vi "getIntersectionFromBallVelocityAndGoalLine.vi"(8 "error in (no error)":errorcluster, 11 "Utilities in":refnum<class "Utilities.lvclass">) -> (0 "error out":errorcluster, 3 "Utilities out":refnum<class "Utilities.lvclass">)   [LabVIEW 2023, in "Utilities.lvclass"]
uses:
  Utilities.lvclass
  Game_class/Game.lvclass
  Game_class/Game.lvclass/Game.ctl
  Ball_class/Ball.lvclass/Ball.ctl
  Object_class/Object.lvclass/Object.ctl
  Game_class/Read BallRef.vi
  Game_class/Read FieldRef.vi
  Ball_class/Read v_x.vi
  Ball_class/Read v_y.vi
  Object_class/Read x.vi
  Object_class/Read y.vi
  Ball_class/Ball.lvclass
  Field_class/Field.lvclass
panel:
  out "y_intersection":dbl
  out "x_intersection":dbl
  in  "Game":refnum<class "Game.lvclass">
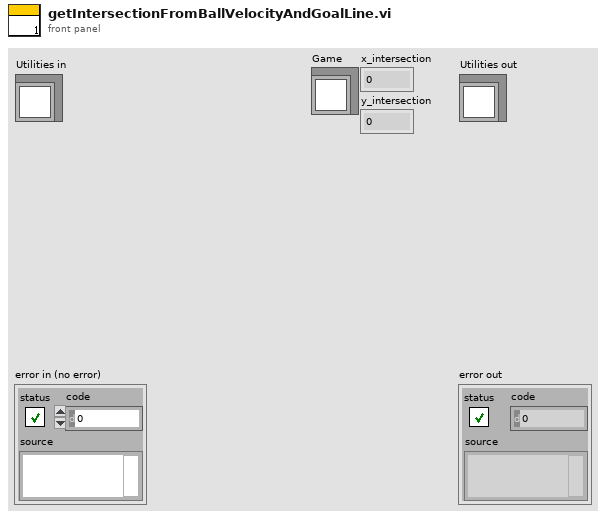
[diagram p1: front panel]
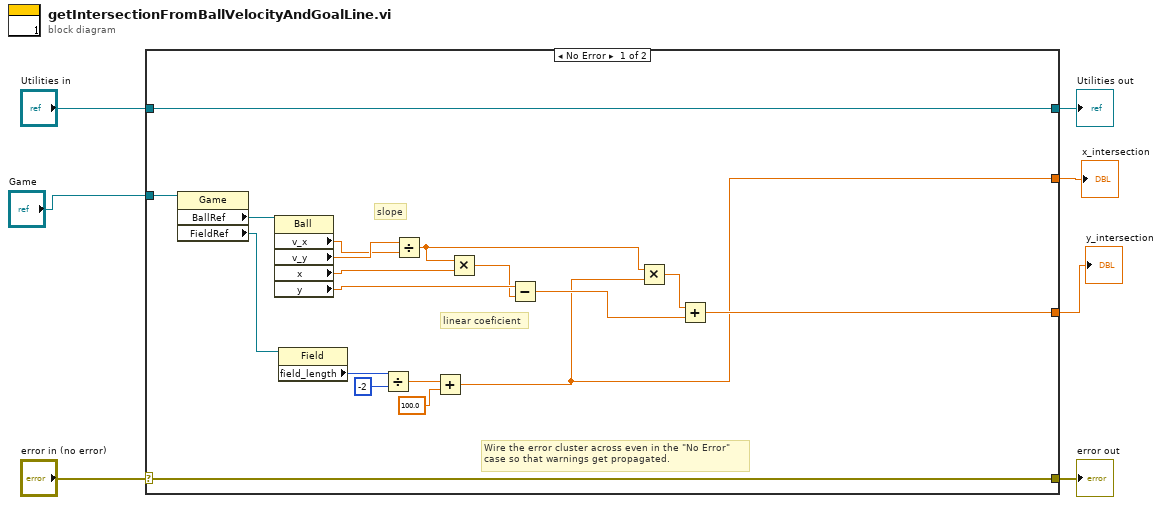
[diagram p0: block diagram]
diagram:
  n1 = case shown="No Error" "error in (no error)" {
    selector: "error in (no error)" -> [w25 w28]
    tunnel: [w25 w28] -> w6
    tunnel: [w26 w27] -> w4
    tunnel: "Utilities in" -> [w26 w27]
    tunnel: "Game" -> [w24 _]
    tunnel: [w9 _] -> w2
    tunnel: [w11 _] -> w1
    frame No Error {
      # "linear coeficient"
      # "slope"
      # "Wire the error cluster across even in the \"No Error\"\ncase so that warnings get propagated."
      n2 = property class="Game"(reference=w24) -> ("BallRef"=w23:refnum<class "Ball.lvclass">, "FieldRef"=w19:refnum<class "Field.lvclass">)  [unwired: 1 in, 2 out]
      n3 = property class="Ball"(reference=w23) -> ("v_x"=w21:dbl, "v_y"=w22:dbl, "x"=w20:dbl, "y"=w16:dbl)  [unwired: 1 in, 2 out]
      n4 = property class="Field"(reference=w19) -> ("field_length"=w18:i32)  [unwired: 1 in, 2 out]
      n5 = Divide(x=w18, y=-2) -> (x/y=w10:dbl)
      n6 = Divide(x=w22, y=w21) -> (x/y=w14:dbl)
      n7 = Add(x=w10, y=100.0) -> (x+y=w9:dbl)
      n8 = Multiply(x=w14, y=w20) -> (x*y=w15:dbl)
      n9 = Subtract(x=w16, y=w15) -> (x-y=w12:dbl)
      n10 = Multiply(x=w14, y=w9) -> (x*y=w13:dbl)
      n11 = Add(x=w13, y=w12) -> (x+y=w11:dbl)
    }
    frame Error {
    }
  }
  "error out" <- w6
  "Utilities out" <- w4
  "x_intersection" <- w2
  "y_intersection" <- w1
